vi "BallToGoalSkillVss.vi"(8 "error in (no error)":errorcluster, 9 "Game":refnum<class "Game.lvclass">, 10 "Robot in":refnum<class "Robot.lvclass">, 11 "BallToGoalSkillVSS in":refnum<class "BallToGoalSkillVSS.lvclass">) -> (0 "error out":errorcluster, 2 "Robot out":refnum<class "Robot.lvclass">, 3 "BallToGoalSkillVSS out":refnum<class "BallToGoalSkillVSS.lvclass">)   [LabVIEW 2023, in "BallToGoalSkillVSS.lvclass"]
uses:
  BallToGoalSkillVSS.lvclass
  Robot_class/Robot.lvclass
  Game_class/Game.lvclass
  Game_class/Game.lvclass/Game.ctl
  Object_class/Object.lvclass/Object.ctl
  Robot_class/Robot.lvclass/Robot.ctl
  Game_class/Read BallRef.vi
  Game_class/Read FieldRef.vi
  Object_class/Read x.vi
  Object_class/Read y.vi
  Robot_class/Write dest_x.vi
  Robot_class/Write dest_y.vi
  Robot_class/Write dest_orientation.vi
  Ball_class/Ball.lvclass
  C:/Users/roboi/Downloads/VSS_AI-Larc2023/Object_class/Object.lvclass
  Field_class/Field.lvclass
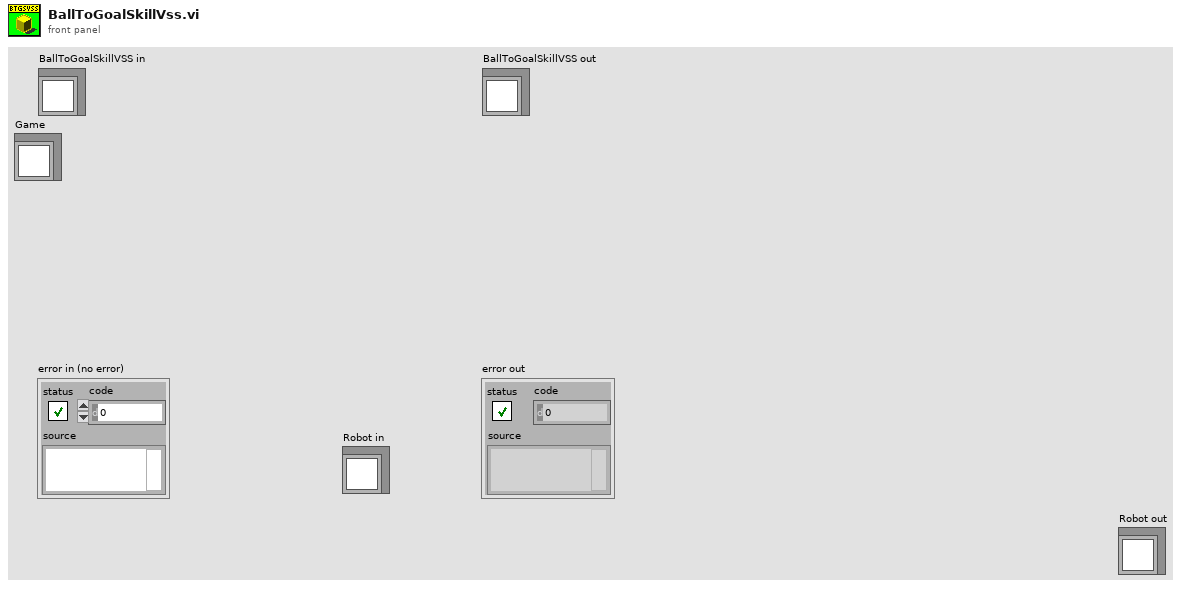
[diagram p1: front panel]
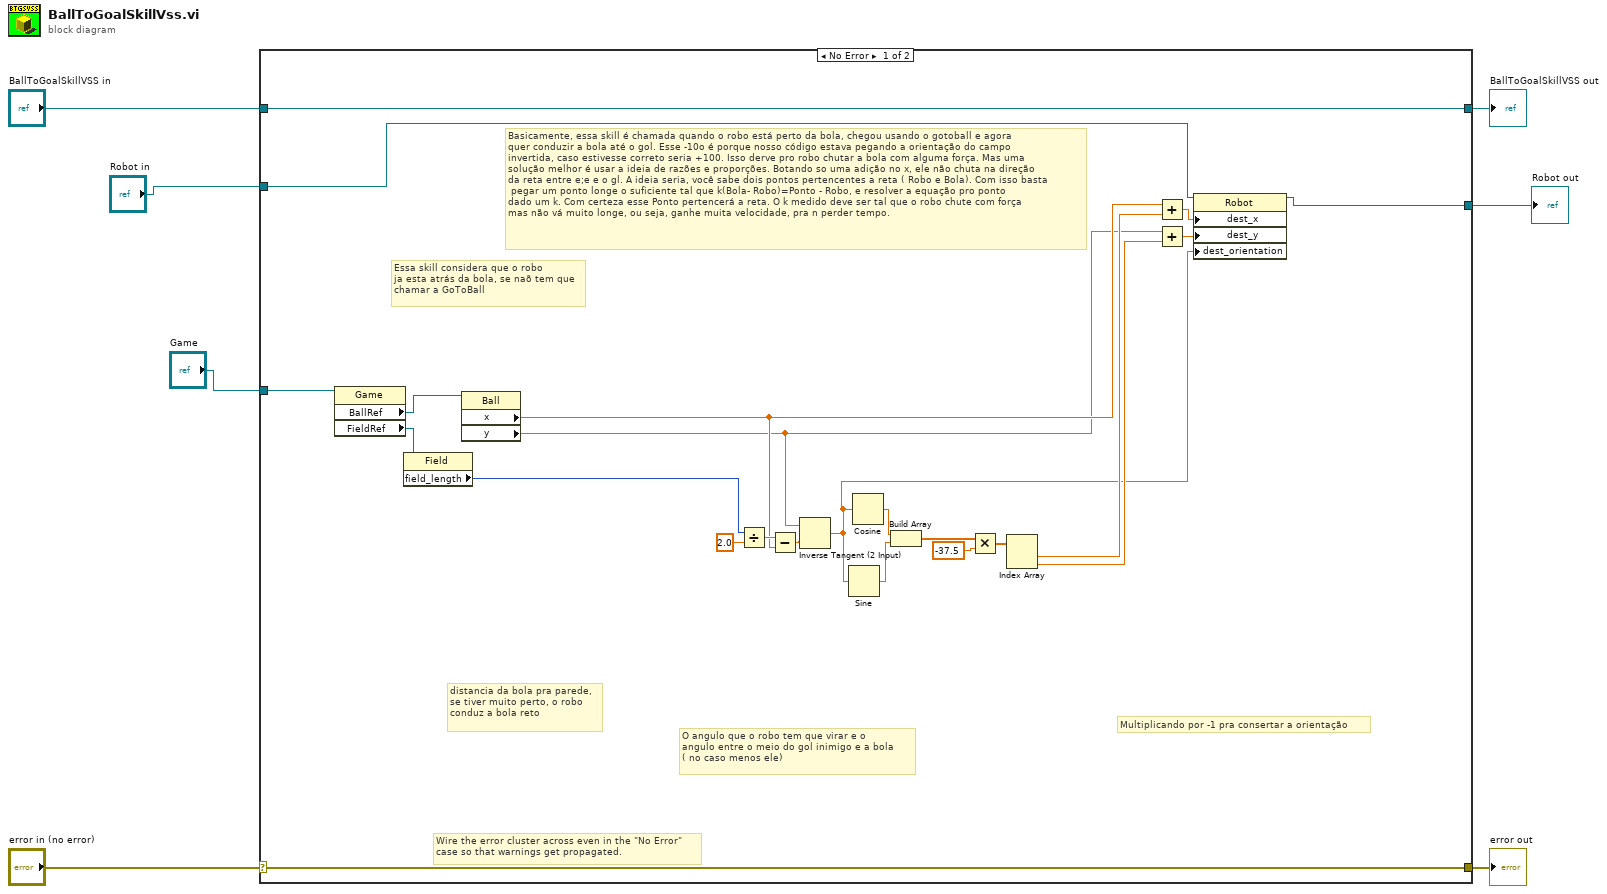
[diagram p0: block diagram]
diagram:
  n1 = case shown="No Error" "error in (no error)" {
    selector: "error in (no error)" -> [w29 w33]
    tunnel: [w29 w33] -> w6
    tunnel: [w30 w32] -> w4
    tunnel: "BallToGoalSkillVSS in" -> [w30 w32]
    tunnel: "Robot in" -> [w28 w31]
    tunnel: [w24 w31] -> w2
    tunnel: "Game" -> [w27 _]
    frame No Error {
      # "Multiplicando por -1 pra consertar a orientação"
      # "O angulo que o robo tem que virar e o\nangulo entre o meio do gol inimigo e a bola\n( no caso menos ele)"
      # "Basicamente, essa skill é chamada quando o robo está perto da bola, chegou usando o gotoball e agora\nquer conduzir a bola até o gol. Esse -10o é porque nosso código estava pegando a orientação do campo \ninvertida, caso estivesse correto seria +100. Isso derve pro robo chutar a bola com alguma força. Mas uma \nsolução melhor é usar a ideia de razões e proporções. Botando so uma adição no x, ele não chuta na direção\nda reta entre e;e e o gl. A ideia seria, você sabe dois pontos pertencentes a reta ( Robo e Bola). Com isso basta \n pegar um ponto longe o suficiente tal que k(Bola- Robo)=Ponto - Robo, e resolver a equação pro ponto\ndado um k. Com certeza esse Ponto pertencerá a reta. O k medido deve ser tal que o robo chute com força\nmas não vá muito longe, ou seja, ganhe muita velocidade, pra n perder tempo."
      # "distancia da bola pra parede, se tiver muito perto, o robo conduz a bola reto"
      # "Essa skill considera que o robo \nja esta atrás da bola, se naõ tem que\nchamar a GoToBall"
      # "Wire the error cluster across even in the \"No Error\"\ncase so that warnings get propagated."
      n2 = property class="Game"(reference=w27) -> ("BallRef"=w26:refnum<class "Ball.lvclass">, "FieldRef"=w25:refnum<class "Field.lvclass">)  [unwired: 1 in, 2 out]
      n3 = property class="Field"(reference=w25) -> ("field_length"=w20:i32)  [unwired: 1 in, 2 out]
      n4 = property class="Ball"(reference=w26) -> ("x"=w13:dbl, "y"=w10:dbl)  [unwired: 1 in, 2 out]
      n5 = Divide(x=w20, y=2.0) -> (x/y=w21:dbl)
      n6 = Subtract(x=w21, y=w13) -> (x-y=w22:dbl)
      n7 = Inverse Tangent (2 Input)(1:w22, 2:w10) -> (0:w8:dbl)
      n8 = Sine(x=w8) -> (sin(x)=w18:dbl)
      n9 = Cosine(x=w8) -> (cos(x)=w19:dbl)
      n10 = Build Array(w19, w18) -> (w17:dbl[])
      n11 = Multiply(x=w17, y=-37.5) -> (x*y=w16:dbl[])
      n12 = Index Array(array=w16) -> (element #1=w14:dbl, element #2=w9:dbl)  [unwired: 2 in]
      n13 = Add(x=w13, y=w14) -> (x+y=w12:dbl)
      n14 = Add(x=w10, y=w9) -> (x+y=w11:dbl)
      n15 = property class="Robot"(reference=w28, "dest_x"=w12, "dest_y"=w11, "dest_orientation"=w8) -> (reference out=w24:refnum<class "Robot.lvclass">)  [unwired: 1 in, 1 out]
    }
    frame Error {
    }
  }
  "error out" <- w6
  "BallToGoalSkillVSS out" <- w4
  "Robot out" <- w2
